vi "_connectSlave.vi"(9 "Boolean in":refnum<vi>, 10 "port":u16, 11 "IP":string) -> (3 "连接与否":bool)   [LabVIEW 2020]
uses:
  global/GlobalVariable.vi
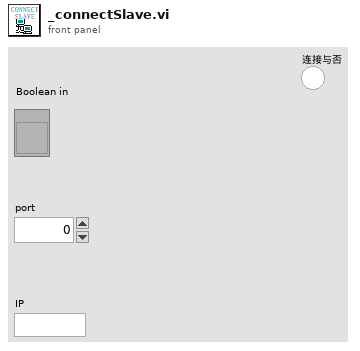
[diagram p1: front panel]
types:
  T1 = enum8{"Enabled", "Disabled", "Disabled and Grayed Out"}
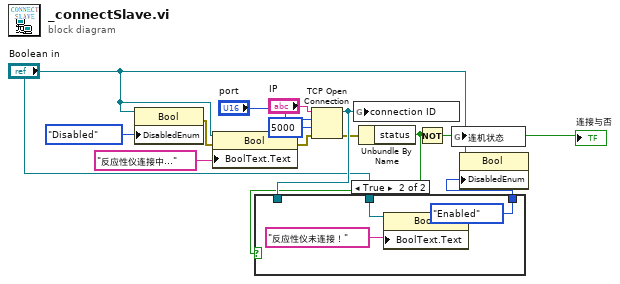
[diagram p0: block diagram]
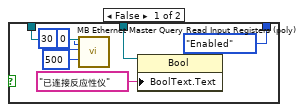
[diagram p2: hidden frame]
diagram:
  n1 = property on="Property Node" class="Bool"(reference="Boolean in", "DisabledEnum"=T1."Disabled" ("Disabled")) -> (error out=w3:errorcluster)  [unwired: 1 in, 1 out]
  n2 = property on="Property Node" class="Bool"(reference="Boolean in", error in=w3, "BoolText.Text"="反应性仪连接中…" ("Boolean Text.Text")) -> (error out=w4:errorcluster)  [unwired: 1 out]
  n3 = TCP Open Connection(address="IP", remote port or service name="port", timeout ms (60000)=5000, error in (no error)=w4) -> (connection ID=w13:refnum<k5>, error out=w12:errorcluster)  [unwired: 1 in]
  n4 = global write "GlobalVariable.vi" "connection ID"(w13) -> ()
  n5 = Unbundle By Name(w12) -> ("status"=w7:bool)
  n6 = case shown="True" w7 {
    tunnel: [T1."Enabled" ("Disabled") T1."Enabled" ("Disabled")] -> w8
    tunnel: w13 -> [w17 _]
    tunnel: "Boolean in" -> [w14 w21]
    frame False {
      n7 = call "MB Ethernet Master Query Read Input Registers (poly).vi"("TCP Connection Refnum in"=w17, "Starting Address"=u16 0, "Quantity"=u16 30, "Timeout"=500) -> ()  [unwired: 12 in, 4 out]
      n8 = property on="Property Node" class="Bool"(reference=w14, "BoolText.Text"="已连接反应性仪") -> ()  [unwired: 1 in, 2 out]
    }
    frame True {
      n9 = property on="Property Node" class="Bool"(reference=w21, "BoolText.Text"="反应性仪未连接！") -> ()  [unwired: 1 in, 2 out]
    }
  }
  n10 = Not(x=w7) -> (.not. x?=w6:bool)
  "连接与否" <- w6
  n11 = global write "GlobalVariable.vi" "连机状态"(w6) -> ()
  n12 = property on="Property Node" class="Bool"(reference="Boolean in", "DisabledEnum"=w8) -> ()  [unwired: 1 in, 2 out]
